vi "is-valid.vi"(11 "UUID in":refnum<class "UUID.lvclass">) -> (2 "is-valid?":bool)   [LabVIEW 2020, in "graph.lvlib" / "UUID.lvclass"]
uses:
  UUID.lvclass
  UUID.lvclass/UUID.ctl
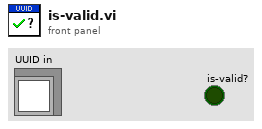
[diagram p1: front panel]
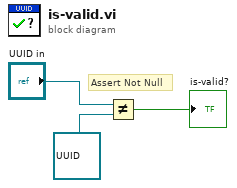
[diagram p0: block diagram]
diagram:
  # "Assert Not Null"
  n1 = Not Equal?(x="UUID in", y=refnum<class "UUID.lvclass"> refnum ("UUID in")) -> (x != y?=→"is-valid?":bool)
